vi "Set Format Units Method.vi"(0 "Display State In":T1, 1 "Units":string, 5 "Precision":i32=3, 7 "s.f. (F) or d.p.(T)":bool, 9 "Container State":T2, 11 "error in (no error)":errorcluster) -> (4 "Display State Out":T1, 15 "error out":errorcluster)   [LabVIEW 2018, in "Waveform Control.xctl"]
uses:
  Waveform Control.xctl
  <vilib>/_xctls/Container State.ctl
  Controls/State.ctl
  Controls/Volatile State Ops.ctl
  <vilib>/_xctls/XControlSupport.lvlib
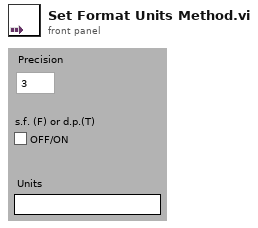
[diagram p1: front panel]
types:
  T1 = typedef "Waveform Control.xctl/State.ctl" = cluster{"Name":string}
  T2 = typedef "XControlSupport.lvlib/Container State.ctl" = cluster{"Indicator?":bool, "Run Mode?":bool, " Refnum":refnum<vi>}
  T3 = typedef "Waveform Control.xctl/Volatile State Ops.ctl" = enum16{"Read", "Write", "Update State from Data"}
  T4 = typedef "Waveform Control.xctl/Waveform State.ctl" = cluster{"Show Axes":bool, "Show Y=0":bool, "Controls":T5, "Show Current Location":bool, "Current Location":i32, "dt":dbl, "t0":timestamp, "Format and Units":string}
  T5 = typedef "Waveform Control.xctl/FP Controls.ctl" = cluster{"Type":T6, "Periods":dbl, "Points":i32, "Offset":dbl, "Amplitdue":dbl, "Phase":dbl, "func":string}
  T6 = typedef "Waveform Control.xctl/Function Types.ctl" = enum16{"Level", "Sine", "Triangle", "Ramp", "Saw Tooth", "Square", "Function"}
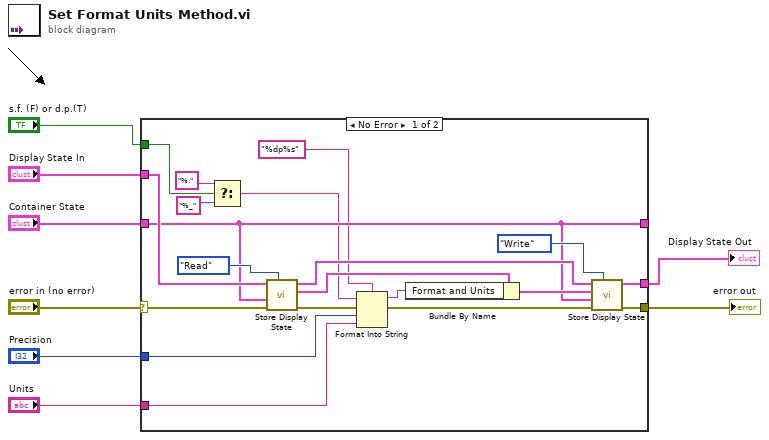
[diagram p0: block diagram]
diagram:
  n1 = case shown="No Error" "error in (no error)" {
    selector: "error in (no error)" -> [w27 w31]
    tunnel: "Display State In" -> [w28 w30]
    tunnel: [w26 w31] -> w2
    tunnel: [w21 w30] -> w1
    tunnel: [w19 w29] -> _
    tunnel: "Container State" -> [w19 w29]
    tunnel: "s.f. (F) or d.p.(T)" -> [w18 _]
    tunnel: "Precision" -> [w13 _]
    tunnel: "Units" -> [w12 _]
    frame No Error {
      n2 = Select(t="%.", s=w18, f="%_") -> (s? t:f=w15:string)
      n3 = call "Store Display State.vi"("Operation In"=Volatile_State_Ops."Read" ("Operation"), "Error In (no Error) In"=w27, "Container State In"=w19, "State In"=w28) -> ("Error Out"=w9:errorcluster, "Waveform State Out"=w24:T4, "Display State Out"=w25:T1)  [unwired: 2 in, 3 out]
      n4 = Format Into String(format string="%dp%s", initial string=w15, error in=w9, w13, w12) -> (resulting string=w11:string, error out=w10:errorcluster)
      n5 = Bundle By Name(cluster=w24, "Format and Units"=w11) -> (w20:T4)
      n6 = call "Store Display State.vi"("Operation In"=Volatile_State_Ops."Write" ("Operation"), "Error In (no Error) In"=w10, "Container State In"=w19, "Waveform State In"=w20, "State In"=w25) -> ("Error Out"=w26:errorcluster, "Display State Out"=w21:T1)  [unwired: 1 in, 4 out]
    }
    frame Error {
    }
  }
  "Display State Out" <- w1
  "error out" <- w2
